vi "StopDebugClient.vi"(5 "error in (no error)":errorcluster) -> (19 "error out":errorcluster)   [LabVIEW 2017, in "G#RemoteProxy.lvclass"]
doc: "Stops then external create process in the background. It is usually stopped when running the garbage collector."
uses:
  G#RemoteProxy.lvclass
  G#Debugger.lvlib
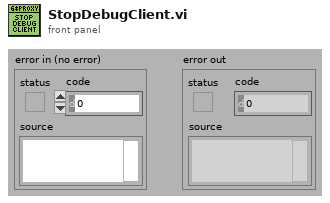
[diagram p1: front panel]
types:
  T1 = enum32{"Bad", "Idle", "Run top level", "Running"}
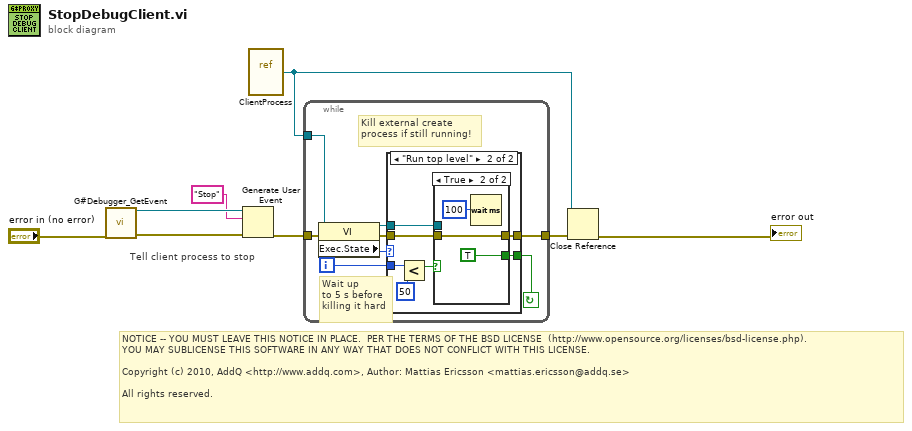
[diagram p0: block diagram]
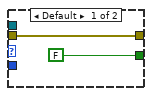
[diagram p2: hidden frame]
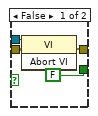
[diagram p3: hidden frame]
diagram:
  # "Tell client process to stop"
  # "NOTICE -- YOU MUST LEAVE THIS NOTICE IN PLACE.  PER THE TERMS OF THE BSD LICENSE  (http://www.opensource.org/licenses/bsd-license.php).\nYOU MAY SUBLICENSE THIS SOFTWARE IN ANY WAY THAT DOES NOT CONFLICT WITH THIS LICENSE.\n\nCopyright (c) 2010, AddQ <http://www.addq.com>, Author: Mattias Ericsson <mattias.ericsson@addq.se>\n\nAll rights reserved."
  n1 = call "G#Debugger_GetEvent.vi"("error in (no error)"="error in (no error)") -> ("Debugger Event"=w2:refnum<user-event>, "error out"=w3:errorcluster)  [unwired: 17 in]
  n2 = Generate User Event(user event=w2, event data cluster="Stop" ("event data"), error in=w3) -> (error out=w4:errorcluster)  [unwired: 1 in, 1 out]
  n3 = vi-ref "ClientProcess.vi"() -> (w6:refnum<vi>)
  n4 = while {
    tunnel: w4 -> [w16]
    tunnel: [w13] -> w7
    tunnel: w6 -> [w11]
    i -> [w9]
    stop <- w10 continue-if-true
    # "Wait up\nto 5 s before\nkilling it hard"
    # "Kill external create\nprocess if still running!"
    n5 = property class="VI"(reference=w11, error in=w16) -> (reference out=w12:refnum<vi>, error out=w14:errorcluster, "Exec.State"=w15:T1)
    n6 = case shown="\"Run top level\"" w15 {
      tunnel: [w18 w21] -> w13
      tunnel: w14 -> [w18 w22]
      tunnel: w12 -> [_ w19]
      tunnel: [FALSE w20] -> w10
      tunnel: w9 -> [_ w25]
      frame Default {
      }
      frame "Run top level" {
        n7 = Less?(x=w25, y=50) -> (x < y?=w23:bool)
        n8 = case shown="True" w23 {
          tunnel: w22 -> [w27 w31]
          tunnel: [w28 w31] -> w21
          tunnel: [FALSE TRUE] -> w20
          tunnel: w19 -> [w26 _]
          frame False {
            n9 = invoke class="VI" method="Abort VI"(reference=w26, error in=w27) -> (error out=w28:errorcluster)  [unwired: 1 in, 2 out]
          }
          frame True {
            n10 = Wait (ms)(milliseconds to wait=u32 100) -> ()  [unwired: 1 out]
          }
        }
      }
    }
  }
  n11 = Close Reference(reference=w6, error in (no error)=w7) -> (error out=→"error out":errorcluster)
